vi "Canread_jetson_R.vi"(1 "배열":T2(array[cluster]), 3 "Control param in":T1) -> (10 "Control param Out":T1)   [LabVIEW 2019]
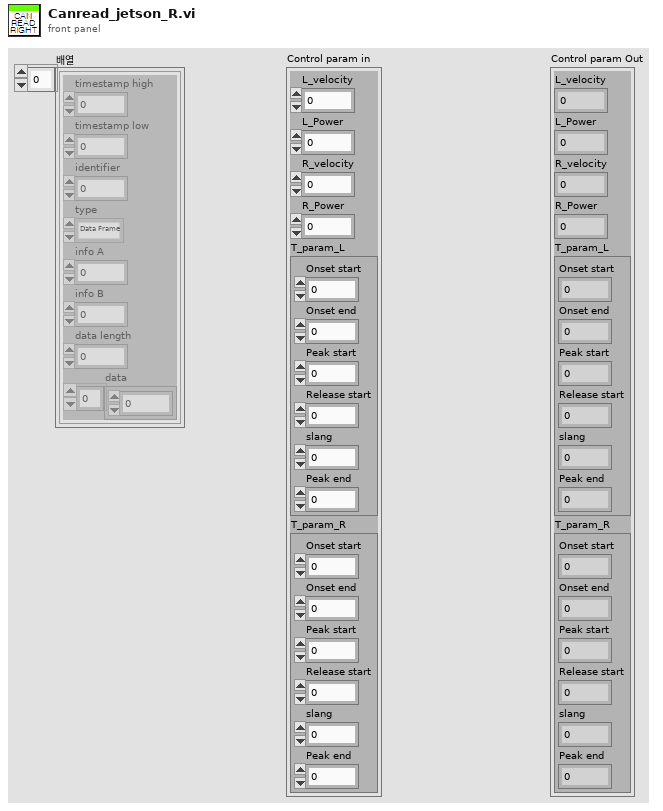
[diagram p1: front panel]
types:
  T1 = cluster{"L_velocity":u32, "L_Power":sgl, "R_velocity":u32, "R_Power":sgl, "T_param_L":cluster{"Onset start":sgl, "Onset end":sgl, "Peak start":sgl, "Release start":sgl, "slang":sgl, "Peak end":sgl}, "T_param_R":cluster{"Onset start":sgl, "Onset end":sgl, "Peak start":sgl, "Release start":sgl, "slang":sgl, "Peak end":sgl}}
  T2 = cluster{"timestamp high":u32, "timestamp low":u32, "identifier":u32, "type":enum8{"Data Frame", "Remote Frame", "(reserved)", "(reserved) ", "(reserved)  ", "(reserved)   ", "Bus Error", "Transceiver Fault"}, "info A":u8, "info B":u8, "data length":u8, "data":u8[]}[]
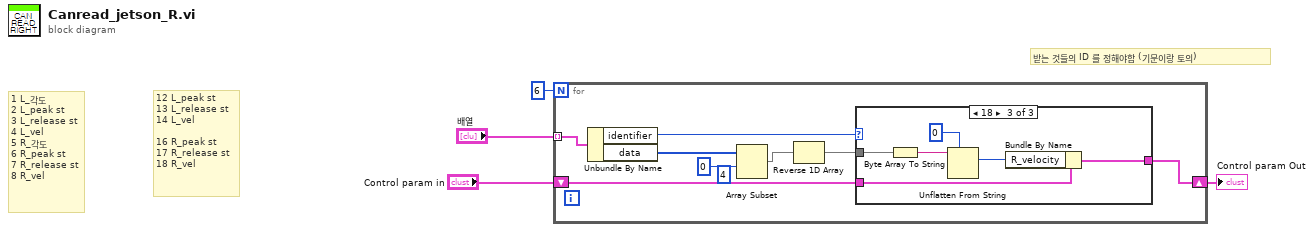
[diagram p0: block diagram]
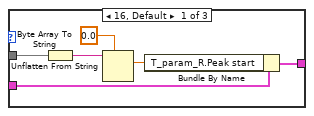
[diagram p2: hidden frame]
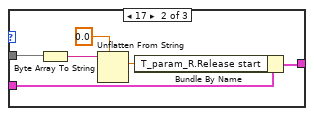
[diagram p3: hidden frame]
diagram:
  # "12 L_peak st\n13 L_release st \n14 L_vel\n\n16 R_peak st\n17 R_release st\n18 R_vel"
  # "받는 것들의 ID 를 정해야함 (기문이랑 토의)"
  # "1 L_각도\n2 L_peak st\n3 L_release st\n4 L_vel\n5 R_각도\n6 R_peak st\n7 R_release st\n8 R_vel"
  n1 = for {
    N: 6 -> [_]
    tunnel: "배열" -> [w12] mode=indexing
    shift-right: [w10] -> w1
    shift-left: "Control param in" -> [w9]
    (unwired) 4 ("길이")
    n2 = Unbundle By Name(w12) -> ("identifier"=w11:u32, "data"=w6:u8[])
    n3 = Array Subset(array=w6, index=0 ("인덱스")) -> (w8:u8[])  [unwired: 1 in]
    n4 = Reverse 1D Array(array=w8) -> (reversed array=w5:u8[])
    n5 = case shown="18" w11 {
      tunnel: w5 -> [w18 w21 w27]
      tunnel: [w14 w20 w26] -> w10
      tunnel: w9 -> [w13 w19 w25]
      frame 16, Default {
        n6 = Byte Array To String(unsigned byte array=w18) -> (string=w17:string)
        n7 = Unflatten From String(type=sgl 0.0, binary string=w17) -> (value=w15:sgl)  [unwired: 3 in, 2 out]
        n8 = Bundle By Name(cluster=w13, "T_param_R.Peak start"=w15) -> (w14:T1)
      }
      frame 17 {
        n9 = Byte Array To String(unsigned byte array=w21) -> (string=w24:string)
        n10 = Unflatten From String(type=sgl 0.0, binary string=w24) -> (value=w22:sgl)  [unwired: 3 in, 2 out]
        n11 = Bundle By Name(cluster=w19, "T_param_R.Release start"=w22) -> (w20:T1)
      }
      frame 18 {
        n12 = Byte Array To String(unsigned byte array=w27) -> (string=w30:string)
        n13 = Unflatten From String(type=u32 0, binary string=w30) -> (value=w28:u32)  [unwired: 3 in, 2 out]
        n14 = Bundle By Name(cluster=w25, "R_velocity"=w28) -> (w26:T1)
      }
    }
  }
  "Control param Out" <- w1
